vi "Driving with the Limelight.vi"() -> (0 "TurnCommand":dbl(knob)=nan scale=-1.0..1.0, 1 "SpeedCommand":dbl(knob)=-0.0 scale=0.0..1.0, 3 "TargetValid":bool)   [LabVIEW 2019]
uses:
  Framework/Robot Global Data.vi
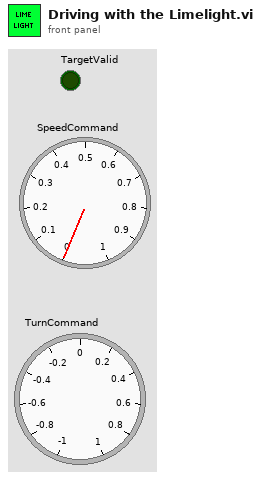
[diagram p1: front panel]
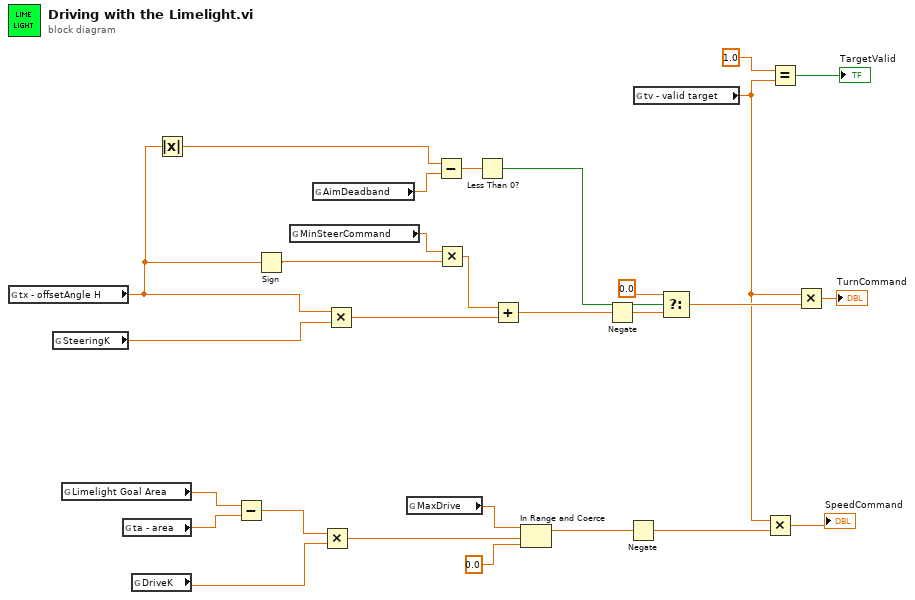
[diagram p0: block diagram]
diagram:
  n1 = global read "Robot Global Data.vi" "tx - offsetAngle H"() -> (w10:dbl)
  n2 = global read "Robot Global Data.vi" "SteeringK"() -> (w4:dbl)
  n3 = global read "Robot Global Data.vi" "Limelight Goal Area"() -> (w5:dbl)
  n4 = global read "Robot Global Data.vi" "ta - area"() -> (w9:dbl)
  n5 = global read "Robot Global Data.vi" "DriveK"() -> (w6:dbl)
  n6 = Absolute Value(x=w10) -> (abs(x)=w25:dbl)
  n7 = Subtract(x=w5, y=w9) -> (x-y=w19:dbl)
  n8 = Sign(1:w10) -> (0:w20:dbl)
  n9 = global read "Robot Global Data.vi" "MinSteerCommand"() -> (w2:dbl)
  n10 = global read "Robot Global Data.vi" "AimDeadband"() -> (w3:dbl)
  n11 = Multiply(x=w19, y=w6) -> (x*y=w18:dbl)
  n12 = Multiply(x=w10, y=w4) -> (x*y=w23:dbl)
  n13 = global read "Robot Global Data.vi" "MaxDrive"() -> (w7:dbl)
  n14 = Subtract(x=w25, y=w3) -> (x-y=w26:dbl)
  n15 = Multiply(x=w2, y=w20) -> (x*y=w24:dbl)
  n16 = Less Than 0?(x=w26) -> (x < 0?=w27:bool)
  n17 = Add(x=w24, y=w23) -> (x+y=w13:dbl)
  n18 = In Range and Coerce(upper limit=w7, x=w18, lower limit=0.0) -> (coerced(x)=w15:dbl)  [unwired: 1 out]
  n19 = Negate(x=w13) -> (-x=w1:dbl)
  n20 = Negate(x=w15) -> (-x=w14:dbl)
  n21 = global read "Robot Global Data.vi" "tv - valid target"() -> (w8:dbl)
  n22 = Select(t=0.0, s=w27, f=w1) -> (s? t:f=w22:dbl)
  n23 = Multiply(x=w8, y=w14) -> (x*y=→"SpeedCommand":dbl)
  n24 = Equal?(x=1.0, y=w8) -> (x = y?=→"TargetValid":bool)
  n25 = Multiply(x=w8, y=w22) -> (x*y=→"TurnCommand":dbl)
